vi "Cannon Global.vi"() -> ()   [LabVIEW 2013]
uses:
  <vilib>/Rock Robotics/WPI/Relay/WPI_RelayValue.ctl
panel:
  in  "Bottom Angle":dbl
  in  "Min Voltage":dbl
  in  "Max Voltage":dbl
  in  "Min Angle":dbl
  in  "Max Angle":dbl
  in  "Cannon Info":T2
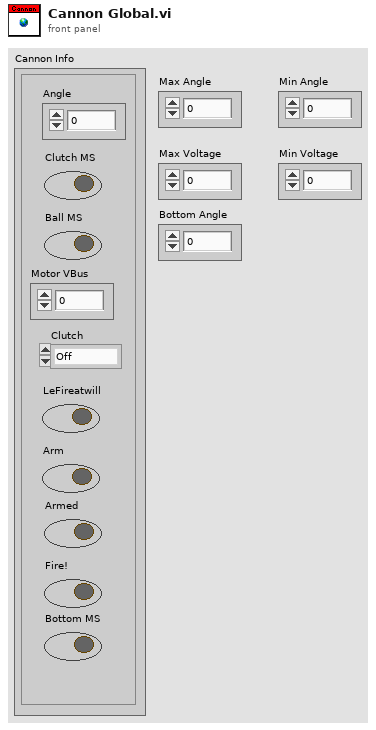
[diagram p1: front panel]
types:
  T1 = typedef "WPI_RelayValue.ctl" = enum16{"Off", "On", "Forward", "Reverse"}
  T2 = cluster{"Angle":dbl, "Clutch MS":bool, "Ball MS":bool, "Clutch ":T1, "LeFireatwill":bool, "Arm":bool, "Armed":bool, "Fire!":bool, "Bottom MS":bool, "Motor VBus":dbl}
diagram:
